vi "_PC_Spectrafilter filter_data_reference.vi"(5 "sn max":dbl, 7 "sn min":dbl, 8 "error in (no error)":errorcluster, 10 "s/n ratio array":dbl[](array[numeric]), 11 "file ref array":path[](array[path])) -> (0 "error out":errorcluster, 3 "new file ref array":path[](array[path]))   [LabVIEW 2018]
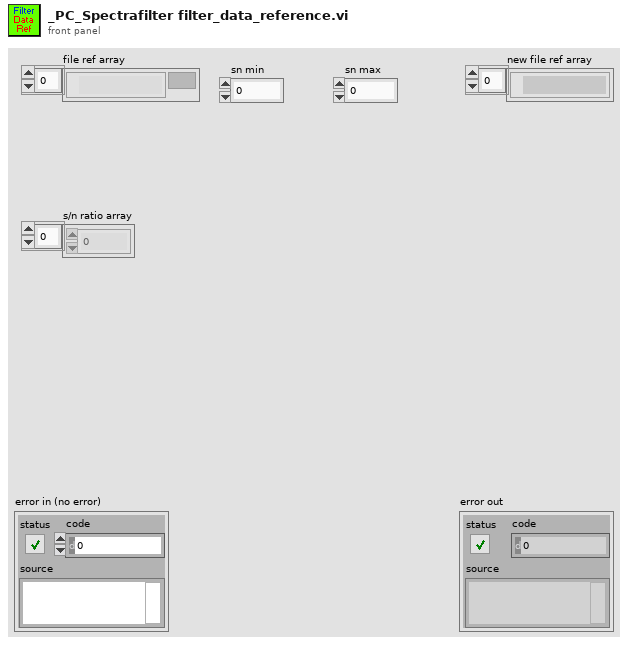
[diagram p1: front panel]
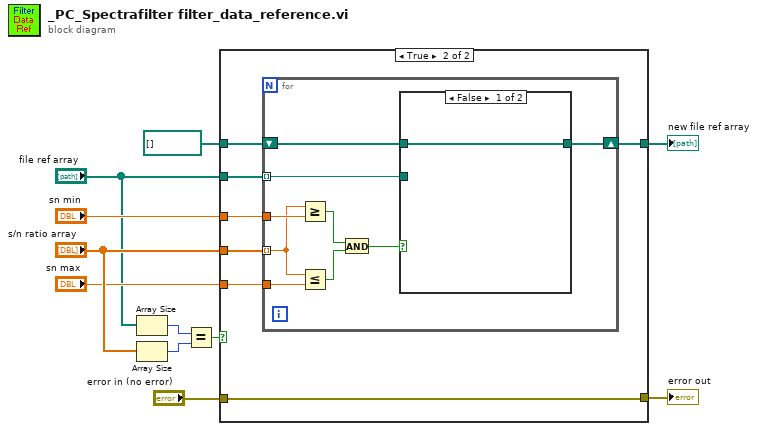
[diagram p0: block diagram]
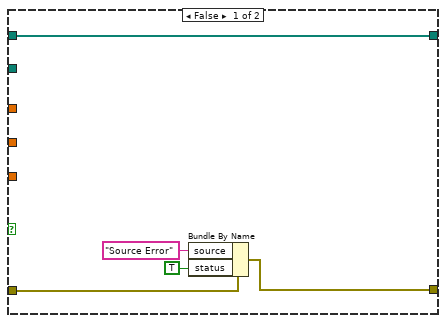
[diagram p2: hidden frame]
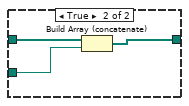
[diagram p3: hidden frame]
diagram:
  n1 = Array Size(array="file ref array") -> (size(s)=w11:i32)
  n2 = Array Size(array="s/n ratio array") -> (size(s)=w10:i32)
  n3 = Equal?(x=w11, y=w10) -> (x = y?=w9:bool)
  n4 = case shown="True" w9 {
    tunnel: "error in (no error)" -> [w16 w18]
    tunnel: "s/n ratio array" -> [_ w22]
    tunnel: "sn max" -> [_ w20]
    tunnel: "sn min" -> [_ w21]
    tunnel: [w13 w18] -> w4
    tunnel: "file ref array" -> [_ w23]
    tunnel: path[] [] ("file ref array") -> [w12 w19]
    tunnel: [w12 w17] -> w1
    frame False {
      n5 = Bundle By Name(cluster=w16, "source"="Source Error", "status"=TRUE) -> (w13:errorcluster)
    }
    frame True {
      n6 = for {
        tunnel: w23 -> [w25] mode=indexing
        tunnel: w22 -> [w31] mode=indexing
        tunnel: w21 -> [w32]
        tunnel: w20 -> [w30]
        shift-right: [w24] -> w17
        shift-left: w19 -> [w26]
        n7 = Greater Or Equal?(x=w31, y=w32) -> (x >= y?=w29:bool)
        n8 = Less Or Equal?(x=w31, y=w30) -> (x <= y?=w28:bool)
        n9 = And(x=w29, y=w28) -> (x .and. y?=w27:bool)
        n10 = case shown="False" w27 {
          tunnel: w26 -> [w33 w36]
          tunnel: w25 -> [_ w35]
          tunnel: [w33 w34] -> w24
          frame False {
          }
          frame True {
            n11 = Build Array (concatenate)(w36, w35) -> (w34:path[])
          }
        }
      }
    }
  }
  "error out" <- w4
  "new file ref array" <- w1
